vi "Update Hardware Configuration File Error.vi"(8 "error in":errorcluster, 11 "Configuration files Ref":T1 format="%.0x") -> (0 "error out":errorcluster, 3 "Configuration files Ref out":T1 format="%.0x")   [LabVIEW 2020, in "Ballard ARINC 429 System Explorer.lvlib" / "Implementation.lvlib"]
uses:
  Implementation.lvlib
  <vilib>/NI VeriStand/Custom Device API/Custom Device Item Ref.ctl
  Scripting/Ballard ARINC 429 Scripting.lvlib
  <vilib>/NI VeriStand/Custom Device API/Custom Device API.lvlib
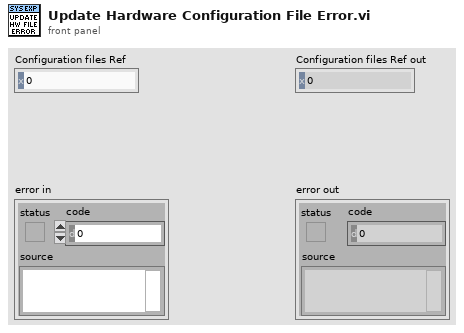
[diagram p1: front panel]
types:
  T1 = typedef "Custom Device API.lvlib/Custom Device Item Ref.ctl" = u64
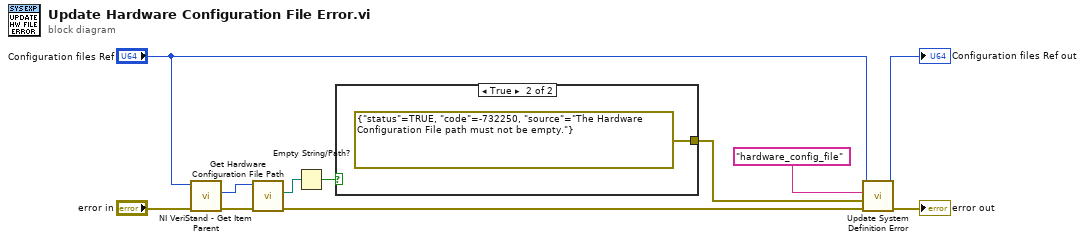
[diagram p0: block diagram]
diagram:
  n1 = call <vilib>:"NI VeriStand - Get Item Parent.vi"("error in (no error)"="error in", "Item Ref in"="Configuration files Ref") -> ("error out"=w3:errorcluster, "Parent Ref"=w2:T1)  [unwired: 6 in, 2 out]
  n2 = call "Get Hardware Configuration File Path.vi"("error in"=w3, "Custom device Ref"=w2) -> ("error out"=w8:errorcluster, "Path"=w5:path)  [unwired: 6 in, 2 out]
  n3 = Empty String/Path?(string/path=w5) -> (empty?=w9:bool)
  n4 = case shown="True" w9 {
    tunnel: [_ errorcluster {"status"=TRUE, "code"=-732250, "source"="The Hardware Configuration File path must not be empty."} ("New Error")] -> w7
    frame False {
    }
    frame True {
    }
  }
  n5 = call "Update System Definition Error.vi"("error to report"=w8, "error in"=w7, "error key"="hardware_config_file", "Configuration files Ref"="Configuration files Ref") -> ("error out"=→"error out":errorcluster, "Configuration files Ref out"=→"Configuration files Ref out":T1)  [unwired: 6 in]
